vi "WaveForms.vi"() -> (0 "2D Double Array 2":i32[][](array[numeric]), 2 "Waveform Chart 3":waveform(i32)[](graph) caption="Waveform Chart 2", 3 "Waveform Chart":waveform(i32)(graph))   [LabVIEW 2023]
panel:
  out "XY Graph":cluster{i32[], u64[]}(graph)
  out "2D Double Array":i32[](array[numeric])
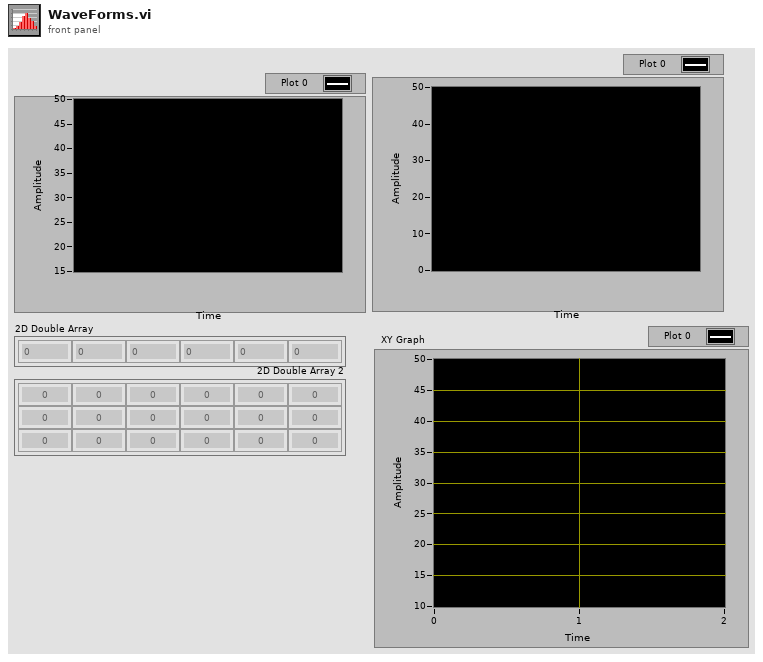
[diagram p1: front panel]
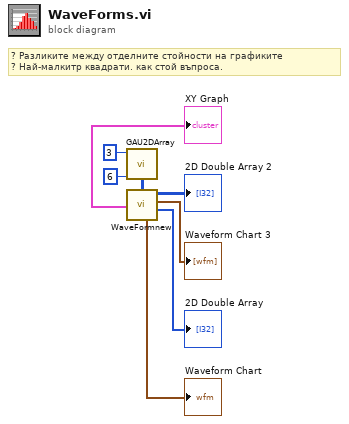
[diagram p0: block diagram]
diagram:
  # "? Разликите между отделните стойности на графиките\n? Най-малкитр квадрати. как стой въпроса."
  n1 = call "GAU2DArray.vi"("Colums"=6, "Rows"=3) -> ("2D Double Array"=w7:i32[][])  [unwired: 8 in, 1 out]
  n2 = call "WaveFormnew.vi"("2D Double Array 3"=w7) -> ("2D Double Array"=→"2D Double Array":i32[], "Waveform Chart 3"=→"Waveform Chart 3":waveform(i32)[], "2D Double Array 2"=→"2D Double Array 2":i32[][], "Waveform Chart"=→"Waveform Chart":waveform(i32), "XY Graph"=→"XY Graph":cluster{i32[], u64[]})  [unwired: 6 in]
